vi "SUB-ONE_Buffer.vi"(7 "mode":enum16{"write", "read"}(ring), 11 "IN":dbl format="%#.6g") -> (3 "OUT":dbl format="%#.6g")   [LabVIEW 2015]
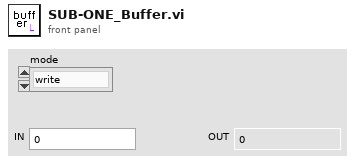
[diagram p1: front panel]
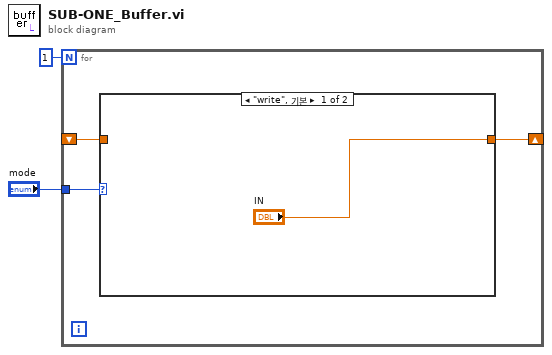
[diagram p0: block diagram]
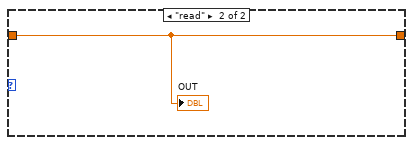
[diagram p2: hidden frame]
diagram:
  n1 = for {
    N: 1 -> [_]
    tunnel: "mode" -> [w5]
    shift-right: [w4] -> _
    shift-left: _ -> [w3]
    n2 = case shown="\"write\", 기본" w5 {
      tunnel: ["IN" w7] -> w4
      tunnel: w3 -> [_ w7]
      frame "write", Default {
      }
      frame "read" {
        "OUT" <- w7
      }
    }
  }
